vi "8（串口数据接收）.vi"() -> ()   [LabVIEW 2017]
uses:
  <vilib>/Instr/_visa.llb/VISA Configure Serial Port (Instr).vi
panel:
  in  "停止":bool
  out "波形图表":dbl(graph)
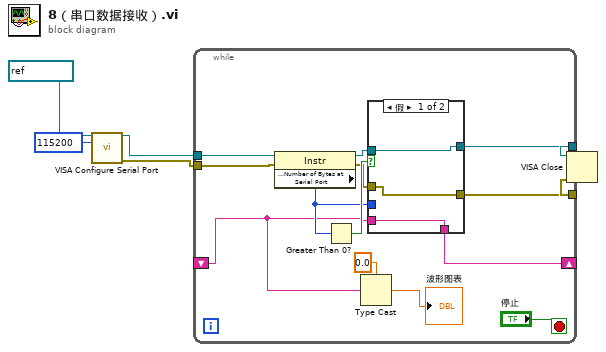
[diagram p0: block diagram]
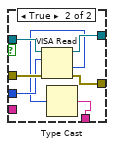
[diagram p2: hidden frame]
diagram:
  n1 = call-poly "VISA Configure Serial Port"("VISA resource name"=refnum<visa-resource-name> "COM2", "baud rate (9600)"=u32 115200) -> ("VISA resource name out"=w4:refnum<visa-resource-name>, "error out"=w3:errorcluster)  [unwired: 12 in]
  n2 = while {
    tunnel: w4 -> [w19]
    tunnel: w3 -> [w18]
    tunnel: [w13] -> w2
    tunnel: [w12] -> w1
    shift-right: [w11] -> _
    shift-left: _ -> [w9]
    stop <- "停止" stop-if-true
    n3 = property class="Instr"(reference=w19, error in=w18) -> (reference out=w16:refnum<visa-resource-name>, error out=w15:errorcluster, "Serial Settings:Number of Bytes at Serial Port"=w14:u32)
    n4 = Greater Than 0?(x=w14) -> (x > 0?=w17:bool)
    n5 = Type Cast(type=0.0, x=w9) -> (*(type *) &x=→"波形图表":dbl)
    n6 = case shown="假" w17 {
      tunnel: w16 -> [w20 w29]
      tunnel: w15 -> [w21 w28]
      tunnel: w14 -> [_ w27]
      tunnel: [w20 w26] -> w13
      tunnel: [w21 w25] -> w12
      tunnel: [w22 w23] -> w11
      tunnel: w9 -> [w22 _]
      frame False {
      }
      frame True {
        n7 = VISA Read(VISA resource name=w29, byte count=w27, error in (no error)=w28) -> (VISA resource name out=w26:refnum<visa-resource-name>, return count=w24:u32, error out=w25:errorcluster)  [unwired: 1 out]
        n8 = Type Cast(x=w24) -> (*(type *) &x=w23:string)  [unwired: 1 in]
      }
    }
  }
  n9 = VISA Close(VISA resource name=w2, error in (no error)=w1) -> ()  [unwired: 1 out]
